vi "GetCharacter.vi"(8 "error in (no error)":errorcluster, 9 "Font":T1={"Font Name:"="", "Size"=12, "Strikeout?"=FALSE, "Italic?"=FALSE, "Underline?"=FALSE, "Outline?"=FALSE, "Shadow?"=FALSE, "Bold?"=FALSE}, 10 "Text Color":u32(colorbox), 11 "Char":string) -> (0 "error out":errorcluster, 3 "Character":refnum<class "Character.lvclass">)   [LabVIEW 2012, in "GlyphFactory.lvclass"]
uses:
  GlyphFactory.lvclass
  Character_class/Character.lvclass
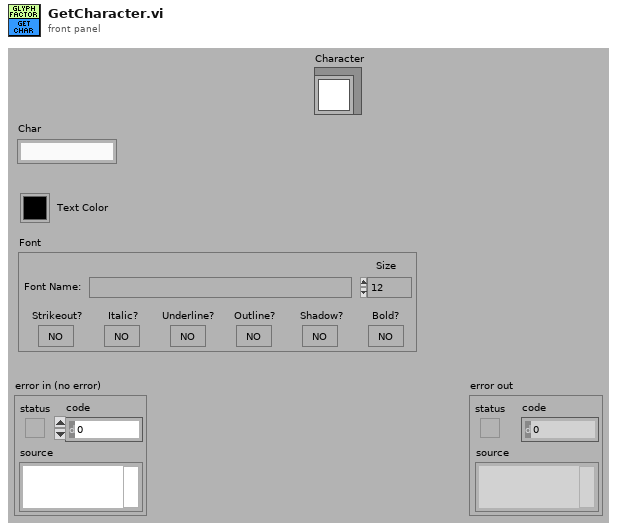
[diagram p1: front panel]
types:
  T1 = cluster{"Font Name:":string, "Size":i16, "Strikeout?":bool, "Italic?":bool, "Underline?":bool, "Outline?":bool, "Shadow?":bool, "Bold?":bool}
  T2 = typedef "GlyphFactory.lvclass/ObjectAttributes.ctl" = cluster{"CharObjectTypes":cluster{"Char":string, "Text Color":u32, "Font":cluster{"Font Name:":string, "Size":i16, "Strikeout?":bool, "Italic?":bool, "Underline?":bool, "Outline?":bool, "Shadow?":bool, "Bold?":bool}}[], "CharObjects":refnum<class "Character.lvclass">[]}
  T3 = cluster{"Char":string, "Text Color":u32, "Font":cluster{"Font Name:":string, "Size":i16, "Strikeout?":bool, "Italic?":bool, "Underline?":bool, "Outline?":bool, "Shadow?":bool, "Bold?":bool}}[]
  T4 = cluster{"Char":string, "Text Color":u32, "Font":cluster{"Font Name:":string, "Size":i16, "Strikeout?":bool, "Italic?":bool, "Underline?":bool, "Outline?":bool, "Shadow?":bool, "Bold?":bool}}
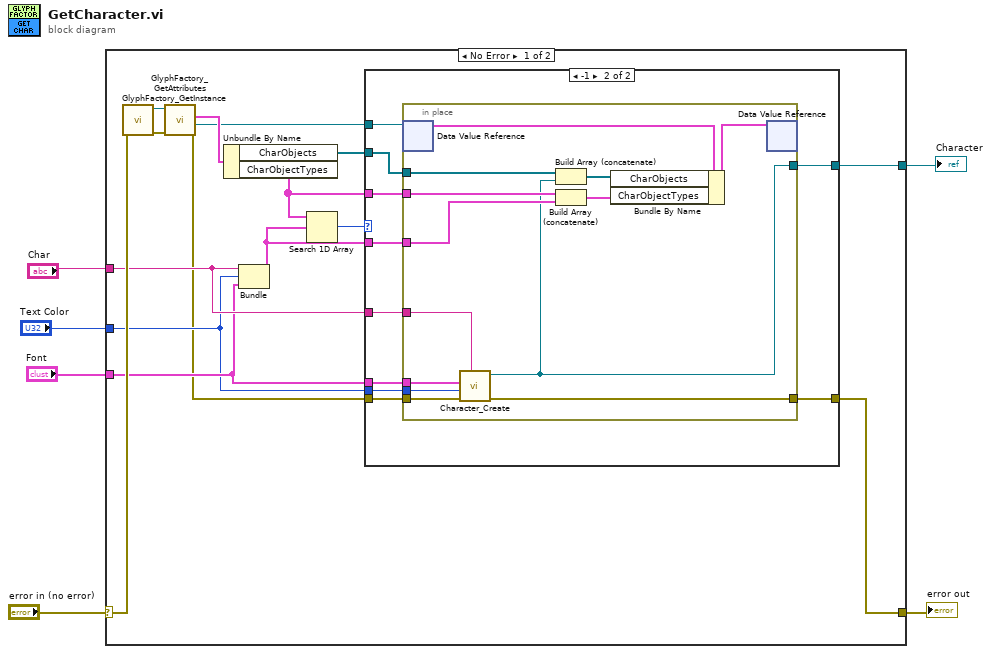
[diagram p0: block diagram]
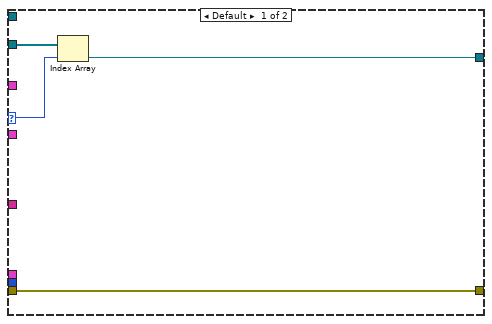
[diagram p2: hidden frame]
diagram:
  n1 = case shown="No Error" "error in (no error)" {
    selector: "error in (no error)" -> [w19 w49]
    tunnel: [w7 w49] -> w5
    tunnel: "Char" -> [w11 _]
    tunnel: "Text Color" -> [w9 _]
    tunnel: "Font" -> [w10 _]
    tunnel: [w15 _] -> w1
    frame No Error {
      n2 = call "GlyphFactory_GetInstance.vi"("error in (no error)"=w19) -> ("error out"=w18:errorcluster, "reference out"=w20:refnum<class "GlyphFactory.lvclass">)  [unwired: 7 in, 2 out]
      n3 = call "GlyphFactory_GetAttributes.vi"("error in (no error)"=w18, "reference in"=w20) -> ("error out"=w8:errorcluster, "DataRef"=w14:refnum<data-value>, "Data"=w21:T2)  [unwired: 6 in, 1 out]
      n4 = Unbundle By Name(w21) -> ("CharObjects"=w16:refnum<class "Character.lvclass">[], "CharObjectTypes"=w13:T3)
      n5 = Bundle("Char"=w11, "Text Color"=w9, "Font"=w10) -> (w12:T4)  [unwired: 1 in]
      n6 = Search 1D Array(1D array=w13, element=w12) -> (index of element=w17:i32)  [unwired: 1 in]
      n7 = case shown="-1" w17 {
        selector: w17 -> [w24 _]
        tunnel: w16 -> [w25 w34]
        tunnel: [w23 w26] -> w15
        tunnel: w14 -> [_ w35]
        tunnel: w13 -> [_ w33]
        tunnel: w12 -> [_ w32]
        tunnel: w8 -> [w22 w31]
        tunnel: w11 -> [_ w30]
        tunnel: w10 -> [_ w29]
        tunnel: w9 -> [_ w28]
        tunnel: [w22 w27] -> w7
        frame Default {
          n8 = Index Array(array=w25, index=w24) -> (element=w23:refnum<class "Character.lvclass">)
        }
        frame -1 {
          n9 = in-place {
            in-place-border: w34 -> [w44]
            in-place-border: w33 -> [w43]
            in-place-border: w32 -> [w42]
            in-place-border: w31 -> [w41]
            in-place-border: w30 -> [w40]
            in-place-border: w29 -> [w39]
            in-place-border: w28 -> [w38]
            in-place-border: [w37] -> w27
            in-place-border: [w36] -> w26
            n10 = in-place-dvr #1(w35) -> (w48:T2)  [unwired: 1 out]
            n11 = call "Character_Create.vi"("Character"=w40, "error in (no error)"=w41, "Color"=w38, "Font"=w39) -> ("error out"=w37:errorcluster, "reference out"=w36:refnum<class "Character.lvclass">)  [unwired: 6 in]
            n12 = Build Array (concatenate)(w44, w36) -> (w46:refnum<class "Character.lvclass">[])
            n13 = Build Array (concatenate)(w43, w42) -> (w45:T3)
            n14 = Bundle By Name(cluster=w48, "CharObjects"=w46, "CharObjectTypes"=w45) -> (w47:T2)
            n15 = in-place-dvr #1(w47) -> ()  [unwired: 2 out]
          }
        }
      }
    }
    frame Error {
    }
  }
  "error out" <- w5
  "Character" <- w1
